vi "SMO.Dictionary.Variant.byValueTestLauncher.vi"() -> ()   [LabVIEW 2013, in "SMO.Dictionary.lvlib" / "SMO.Dictionary.Variant.lvclass"]
uses:
  SMO.Dictionary.Variant.lvclass
  <vilib>/JKI/JKI SMO/SMO/SMO.lvclass/SMO.ctl
  <vilib>/JKI/JKI SMO/SMO/Private/ReftoDVR--SMO.vi
  <vilib>/JKI/JKI SMO/SMO/SMO.lvclass
  SMO.Dictionary/SMO.Dictionary.lvclass
panel:
  out "loop":i32
  out "Events":cluster{"updated":bool, "deleted":bool}
  in  "Delete String":bool
  out "echo":string
  out "Values":variant[](array[variant])
  in  "string":string
  in  "Update String":bool
  out "error out":errorcluster
  in  "Stop":bool
  # "byValue Variant Attributes Dictionary Test"
  # "This example code shows that the dictionary and\nevents work even if the subsystem is not started.\nIf not started, it works synchronously.\nIf started, everything goes through the process."
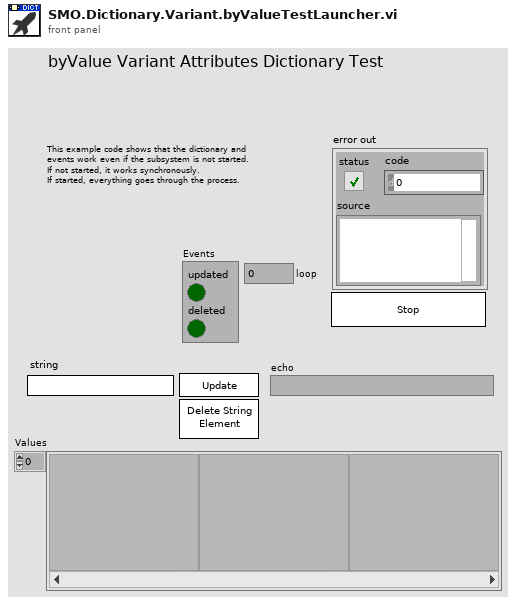
[diagram p1: front panel]
types:
  T1 = typedef "SMO.Dictionary.lvlib/SMO.Dictionary.lvclass/PublicEvents--Cluster.ctl" = cluster{"Cleared":refnum<user-event>, "Deleted":refnum<user-event>, "Updated":refnum<user-event>}
  T2 = cluster{"Event Registration Refnum":refnum<event-registration>}
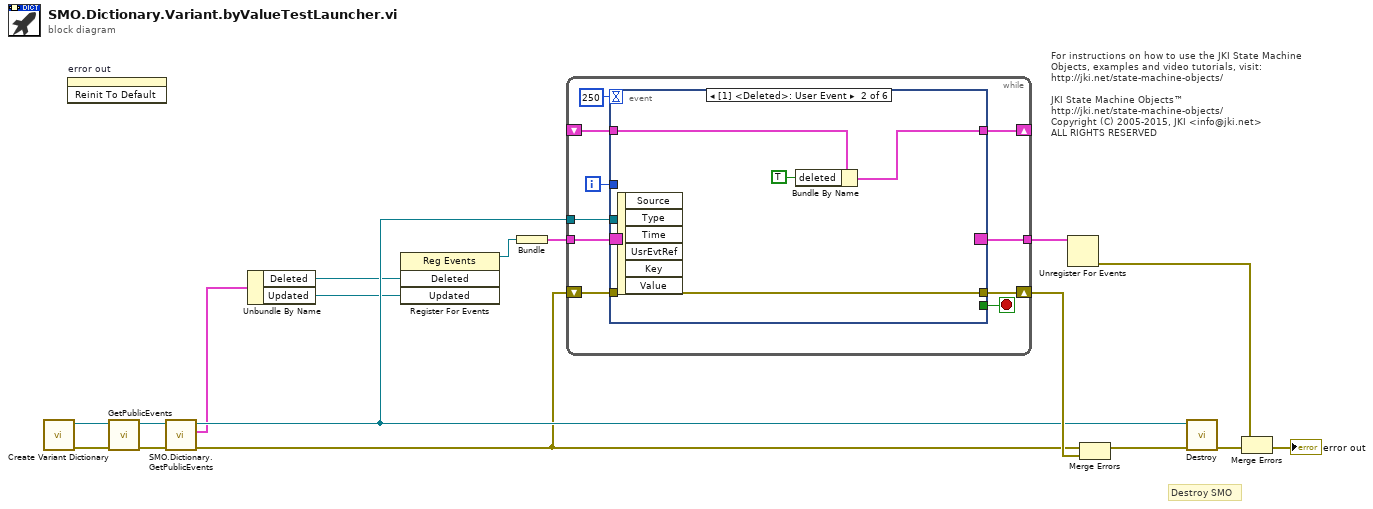
[diagram p0: block diagram]
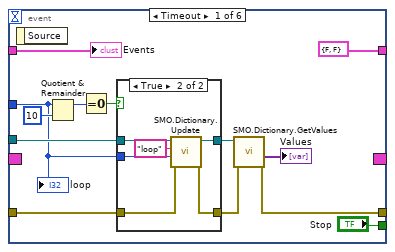
[diagram p2: hidden frame]
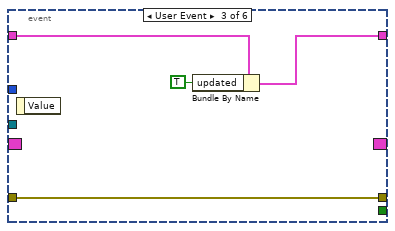
[diagram p4: hidden frame]
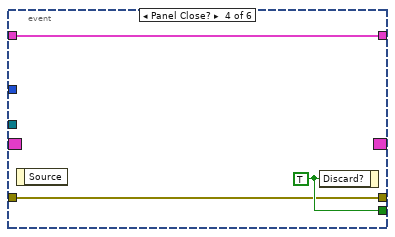
[diagram p5: hidden frame]
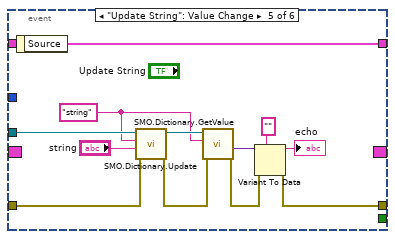
[diagram p6: hidden frame]
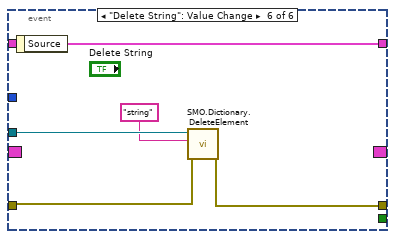
[diagram p7: hidden frame]
diagram:
  # "For instructions on how to use the JKI State Machine Objects, examples and video tutorials, visit:\nhttp://jki.net/state-machine-objects/\n\nJKI State Machine Objects™\nhttp://jki.net/state-machine-objects/\nCopyright (C) 2005-2015, JKI <info@jki.net>\nALL RIGHTS RESERVED"
  # "Destroy SMO"
  n1 = call "Create Variant Dictionary.vi"() -> ("error out"=w6:errorcluster, "SMO.Dictionary.Variant out"=w7:refnum<class "SMO.Dictionary.Variant.lvclass">)  [unwired: 9 in, 1 out]
  n2 = invoke on="error out" class="Clust (strict)" method="Reinit To Default"() -> ()  [unwired: 3 in, 3 out]
  n3 = call <vilib>:"GetPublicEvents.vi"("error in (no error)"=w6, "SMO"=w7) -> ("error out"=w8:errorcluster, "SMO out"=w9:refnum<class "SMO.Dictionary.Variant.lvclass">)  [unwired: 7 in, 1 out]
  n4 = call "SMO.Dictionary.GetPublicEvents.vi"("error in (no error)"=w8, "SMO.Dictionary in"=w9) -> ("error out"=w4:errorcluster, "Public Events"=w3:T1, "SMO.Dictionary out"=w5:refnum<class "SMO.Dictionary.Variant.lvclass">)  [unwired: 7 in]
  n5 = Unbundle By Name(w3) -> ("Deleted"=w2:refnum<user-event>, "Updated"=w1:refnum<user-event>)
  n6 = register-events(w2, w1) -> (reference out=w10:refnum<event-registration>)  [unwired: 2 in, 1 out]
  n7 = Bundle("Event Registration Refnum"=w10) -> (w16:T2)  [unwired: 1 in]
  n8 = while {
    shift-right: [w26] -> w15
    shift-left: w4 -> [w25]
    tunnel: w16 -> [w24]
    tunnel: [w23] -> w17
    tunnel: w5 -> [w22]
    shift-right: [w19] -> _
    shift-left: _ -> [w18]
    i -> [w20]
    stop <- w27 stop-if-true
    n9 = event shown="[1] <Deleted>: User Event" {
      selector: w24 -> [_ _ _ _ _ _]
      dyn-events: [_ _ _ _ _ _] -> w23
      timeout: 250 -> [_ _ _ _ _ _]
      tunnel: ["Stop" _ _ w59 _ _] -> w27
      tunnel: w22 -> [w35 _ _ _ w71 w76]
      tunnel: [w38 w52 w56 w58 w62 w73] -> w26
      tunnel: w25 -> [w33 w52 w56 w58 w70 w74]
      tunnel: w20 -> [w28 _ _ _ _ _]
      tunnel: [cluster{"updated":bool, "deleted":bool} {"updated"=FALSE, "deleted"=FALSE} w49 w53 w57 w60 w72] -> w19
      tunnel: w18 -> [w36 w50 w54 w57 w60 w72]
      event Timeout {
        n10 = event-data() -> ()  [unwired: 1 in, 1 out]
        n11 = Quotient & Remainder(x=w28, y=10) -> (x-y*floor(x/y)=w30:i32)  [unwired: 1 out]
        n12 = Equal To 0?(x=w30) -> (x = 0?=w29:bool)
        n13 = case shown="True" w29 {
          tunnel: w35 -> [w42 w48]
          tunnel: [w42 w47] -> w34
          tunnel: w33 -> [w41 w46]
          tunnel: [w41 w45] -> w32
          tunnel: w28 -> [_ w44]
          frame False {
          }
          frame True {
            n14 = call "SMO.Dictionary.Update.vi"("error in (no error)"=w46, "Value"=w44, "Key (\"\": variant name)"="loop" ("Key (\"\": variant name)"), "SMO.Dictionary"=w48) -> ("error out"=w45:errorcluster, "SMO.Dictionary out"=w47:refnum<class "SMO.Dictionary.Variant.lvclass">)  [unwired: 5 in, 1 out]
          }
        }
        n15 = call "SMO.Dictionary.GetValues.vi"("error in (no error)"=w32, "SMO.Dictionary"=w34) -> ("error out"=w38:errorcluster, "Values"=→"Values":variant[])  [unwired: 5 in, 3 out]
        "Events" <- w36
        "loop" <- w28
      }
      event User Event {
        n16 = event-data() -> ()  [unwired: 1 in, 6 out]
        n17 = Bundle By Name(cluster=w50, "deleted"=TRUE) -> (w49:cluster{"updated":bool, "deleted":bool})
      }
      event User Event {
        n18 = event-data() -> ()  [unwired: 1 in, 1 out]
        n19 = Bundle By Name(cluster=w54, "updated"=TRUE ("deleted")) -> (w53:cluster{"updated":bool, "deleted":bool})
      }
      event Panel Close? {
        w59 = TRUE ("OK")
        n20 = event-data() -> ()  [unwired: 1 in, 1 out]
        n21 = event-data("Discard?"=w59) -> ()  [unwired: 1 in, 1 out]
      }
      event "Update String": Value Change {
        w67 = "string"
        n22 = event-data() -> ()  [unwired: 1 in, 1 out]
        n23 = call "SMO.Dictionary.Update.vi"("error in (no error)"=w70, "Value"="string", "Key (\"\": variant name)"=w67, "SMO.Dictionary"=w71) -> ("error out"=w66:errorcluster, "SMO.Dictionary out"=w68:refnum<class "SMO.Dictionary.Variant.lvclass">)  [unwired: 5 in, 1 out]
        n24 = call "SMO.Dictionary.GetValue.vi"("error in (no error)"=w66, "Key"=w67, "SMO.Dictionary"=w68) -> ("error out"=w63:errorcluster, "Value"=w65:variant)  [unwired: 4 in, 3 out]
        n25 = Variant To Data(error in=w63, type="", Variant=w65) -> (data=→"echo":string, error out=w62:errorcluster)
      }
      event "Delete String": Value Change {
        n26 = event-data() -> ()  [unwired: 1 in, 1 out]
        n27 = call "SMO.Dictionary.DeleteElement.vi"("error in (no error)"=w74, "Key"="string", "SMO.Dictionary"=w76) -> ("error out"=w73:errorcluster)  [unwired: 6 in, 2 out]
      }
    }
  }
  n28 = Unregister For Events(event registration refnum=w17) -> (error out=w14:errorcluster)  [unwired: 1 in]
  n29 = Merge Errors(w4, w15) -> (w11:errorcluster)
  n30 = call <vilib>:"Destroy.vi"("error in (no error)"=w11, "SMO"=w5) -> ("error out"=w12:errorcluster)  [unwired: 9 in]
  n31 = Merge Errors(w14, w12) -> (→"error out":errorcluster)
